vi "Rectangel LineIntersect.vi"(0 "LinePoint1":T1 {"y" format="%.2f"; "x" format="%.2f"}, 1 "LinePoint2":T1 {"y" format="%.2f"; "x" format="%.2f"}, 2 "bounds":T2 {"height" format="%.2f"; "width" format="%.2f"; "y" format="%.2f"; "x" format="%.2f"}, 3 "Margin":i32, 5 "error in (no error)":errorcluster) -> (15 "Intersect":bool, 19 "error out":errorcluster)   [LabVIEW 2014]
doc: "contains"
uses:
  <resource>/Framework/Providers/Open_GDS/UML/General/Point/Point Point2D.ctl
  <resource>/Framework/Providers/Open_GDS/UML/General/Rectangle/Rectangle Rectangle2D.ctl
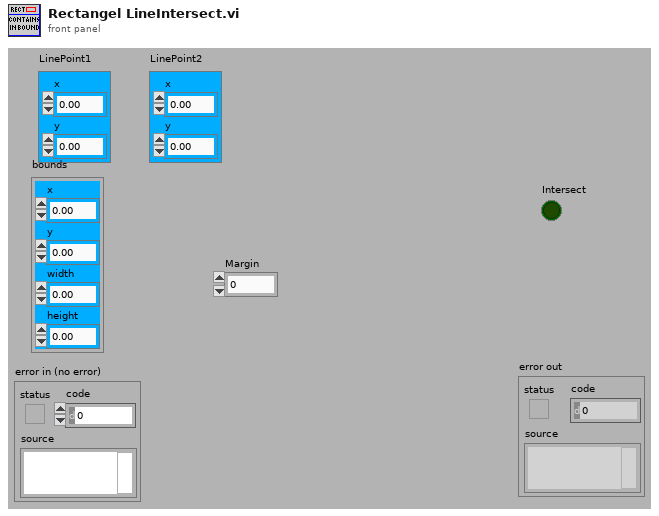
[diagram p1: front panel]
types:
  T1 = typedef "Point Point2D.ctl" = cluster{"x":dbl, "y":dbl}
  T2 = typedef "Rectangle Rectangle2D.ctl" = cluster{"x":dbl, "y":dbl, "width":dbl, "height":dbl}
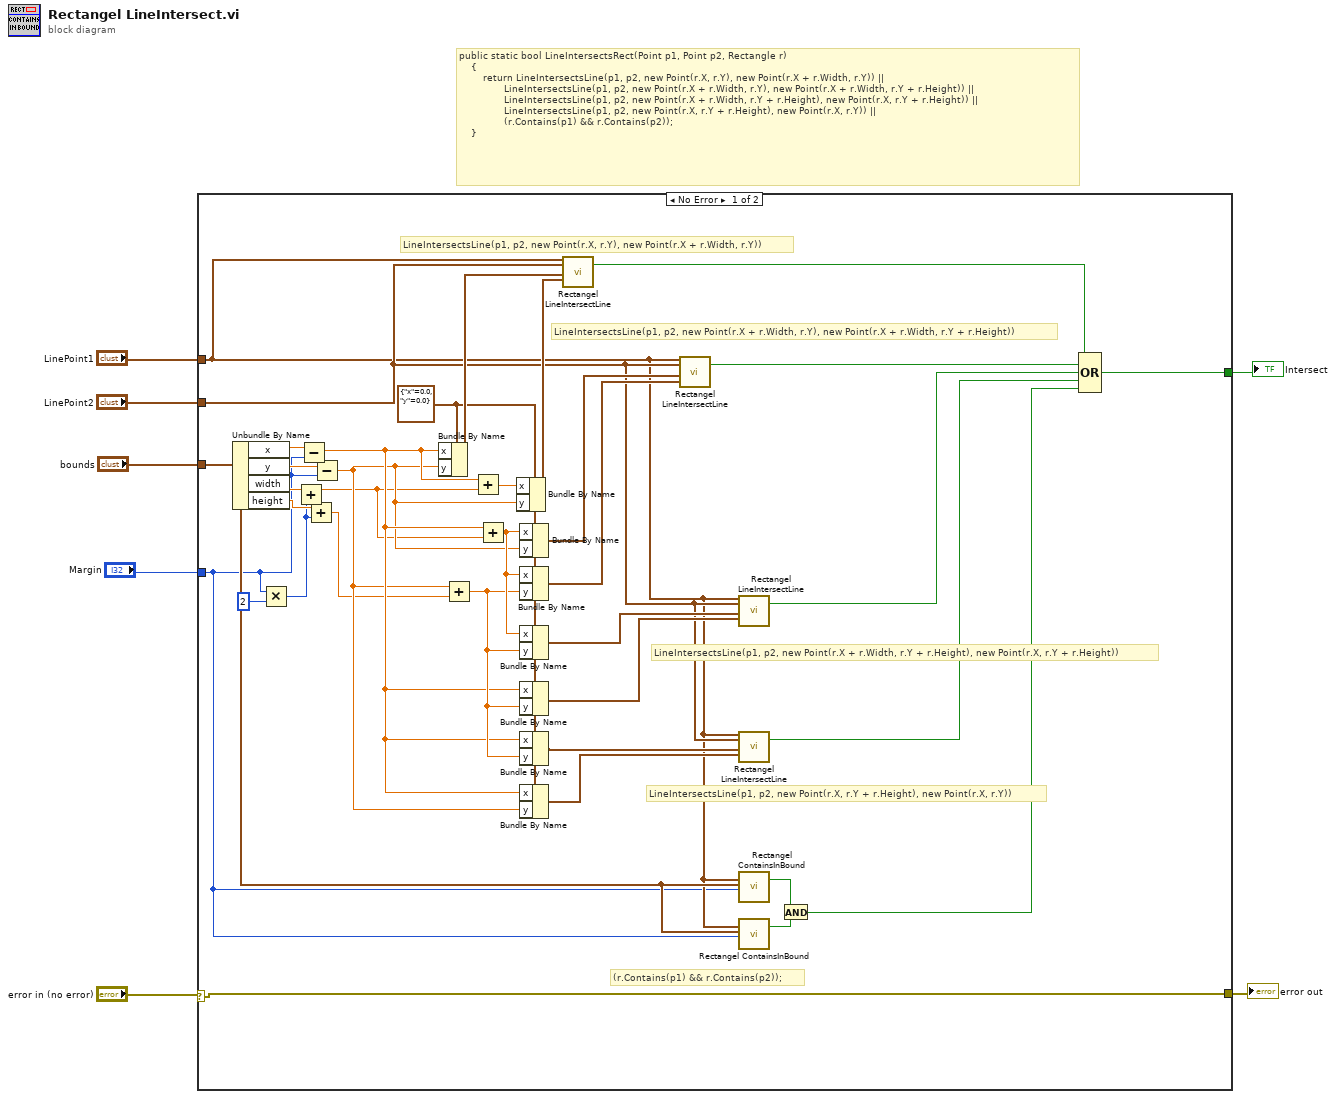
[diagram p0: block diagram]
diagram:
  # "public static bool LineIntersectsRect(Point p1, Point p2, Rectangle r)\n    {\n        return LineIntersectsLine(p1, p2, new Point(r.X, r.Y), new Point(r.X + r.Width, r.Y)) ||\n               LineIntersectsLine(p1, p2, new Point(r.X + r.Width, r.Y), new Point(r.X + r.Width, r.Y + r.Height)) ||\n               LineIntersectsLine(p1, p2, new Point(r.X + r.Width, r.Y + r.Height), new Point(r.X, r.Y + r.Height)) ||\n               LineIntersectsLine(p1, p2, new Point(r.X, r.Y + r.Height), new Point(r.X, r.Y)) ||\n               (r.Contains(p1) && r.Contains(p2));\n    }"
  n1 = case shown="No Error" "error in (no error)" {
    selector: "error in (no error)" -> [w42 w43]
    tunnel: [w42 w43] -> w7
    tunnel: "LinePoint1" -> [w19 _]
    tunnel: "bounds" -> [w20 _]
    tunnel: [w41 _] -> w3
    tunnel: "LinePoint2" -> [w27 _]
    tunnel: "Margin" -> [w8 _]
    frame No Error {
      w26 = T1 {"x"=0.0, "y"=0.0} ("input cluster")
      # "(r.Contains(p1) && r.Contains(p2));"
      # "LineIntersectsLine(p1, p2, new Point(r.X, r.Y + r.Height), new Point(r.X, r.Y))"
      # "LineIntersectsLine(p1, p2, new Point(r.X + r.Width, r.Y + r.Height), new Point(r.X, r.Y + r.Height))"
      # "LineIntersectsLine(p1, p2, new Point(r.X + r.Width, r.Y), new Point(r.X + r.Width, r.Y + r.Height))"
      # "LineIntersectsLine(p1, p2, new Point(r.X, r.Y), new Point(r.X + r.Width, r.Y))"
      n2 = Unbundle By Name(w20) -> ("x"=w25:dbl, "y"=w14:dbl, "width"=w35:dbl, "height"=w34:dbl)
      n3 = Multiply(x=w8, y=2) -> (x*y=w9:i32)
      n4 = Add(x=w35, y=w9) -> (x+y=w12:dbl)
      n5 = Subtract(x=w25, y=w8) -> (x-y=w15:dbl)
      n6 = Add(x=w34, y=w9) -> (x+y=w11:dbl)
      n7 = Subtract(x=w14, y=w8) -> (x-y=w13:dbl)
      n8 = Bundle By Name(cluster=w26, "x"=w15, "y"=w13) -> (w37:T1)
      n9 = Add(x=w13, y=w11) -> (x+y=w24:dbl)
      n10 = Add(x=w15, y=w12) -> (x+y=w39:dbl)
      n11 = Add(x=w15, y=w12) -> (x+y=w32:dbl)
      n12 = Bundle By Name(cluster=w26, "x"=w39, "y"=w13) -> (w38:T1)
      n13 = Bundle By Name(cluster=w26, "x"=w32, "y"=w13) -> (w36:T1)
      n14 = Bundle By Name(cluster=w26, "x"=w32, "y"=w24) -> (w33:T1)
      n15 = Bundle By Name(cluster=w26, "x"=w32, "y"=w24) -> (w31:T1)
      n16 = Bundle By Name(cluster=w26, "x"=w15, "y"=w24) -> (w30:T1)
      n17 = Bundle By Name(cluster=w26, "x"=w15, "y"=w24) -> (w23:T1)
      n18 = Bundle By Name(cluster=w26, "x"=w15, "y"=w13) -> (w22:T1)
      n19 = call <resource>:"Rectangel LineIntersectLine.vi"("LineA-Point1(l1p1)"=w19, "LineA-Point2(l1p2)"=w27, "LineB-Point1(l2p1)"=w37, "LineB-Point2(l2p2)"=w38) -> ("Intersect"=w40:bool)  [unwired: 14 in, 1 out]
      n20 = call <resource>:"Rectangel LineIntersectLine.vi"("LineA-Point1(l1p1)"=w19, "LineA-Point2(l1p2)"=w27, "LineB-Point1(l2p1)"=w36, "LineB-Point2(l2p2)"=w33) -> ("Intersect"=w29:bool)  [unwired: 14 in, 1 out]
      n21 = call <resource>:"Rectangel LineIntersectLine.vi"("LineA-Point1(l1p1)"=w19, "LineA-Point2(l1p2)"=w27, "LineB-Point1(l2p1)"=w31, "LineB-Point2(l2p2)"=w30) -> ("Intersect"=w28:bool)  [unwired: 14 in, 1 out]
      n22 = call <resource>:"Rectangel LineIntersectLine.vi"("LineA-Point1(l1p1)"=w19, "LineA-Point2(l1p2)"=w27, "LineB-Point1(l2p1)"=w23, "LineB-Point2(l2p2)"=w22) -> ("Intersect"=w21:bool)  [unwired: 14 in, 1 out]
      n23 = call <resource>:"Rectangel ContainsInBound.vi"("point2D"=w19, "bounds"=w20, "AdditionalMargin"=w8) -> ("contains"=w18:bool)  [unwired: 15 in, 1 out]
      n24 = call <resource>:"Rectangel ContainsInBound.vi"("point2D"=w19, "bounds"=w20, "AdditionalMargin"=w8) -> ("contains"=w17:bool)  [unwired: 15 in, 1 out]
      n25 = And(x=w18, y=w17) -> (x .and. y?=w16:bool)
      n26 = Compound Arithmetic op=OR(w40, w29, w28, w21, w16) -> (w41:bool)
    }
    frame Error {
    }
  }
  "error out" <- w7
  "Intersect" <- w3
